vi "sort_scan_settings.vi"(7 "Scan settings array":T1[](array[typedef]) {"Enable display" items=["False", "True"]; "Current range" items=["Auto", "1 uA", "10 uA", "100 uA", "1 mA", "10 mA", "100 mA", "1 A"]; "Integration time (ms)" min=0.2; "Auto settling delay" items=["False", "True"]; "Sweep mode" items=["Staircase", "Pulsed"]; "Electrode configuration" items=["2-wire", "4-wire"]; "Logarithmic sweep" items=["False", "True"]; "Repeat scans" items=["False", "True"]; "No. of repeat scans" min=1.0 step=1.0; "Stabilisation mode" items=["V", "I"]; "Dual sweep" items=["False", "True"]; "Settling delay (ms)" min=0.0}, 10 "Setting name array":string[](array[string])) -> (0 "Sorted settings array":T1[](array[typedef]) {"Enable display" items=["False", "True"]; "Current range" items=["Auto", "1 uA", "10 uA", "100 uA", "1 mA", "10 mA", "100 mA", "1 A"]; "Integration time (ms)" min=0.2; "Auto settling delay" items=["False", "True"]; "Sweep mode" items=["Staircase", "Pulsed"]; "Electrode configuration" items=["2-wire", "4-wire"]; "Logarithmic sweep" items=["False", "True"]; "Repeat scans" items=["False", "True"]; "No. of repeat scans" min=1.0 step=1.0; "Stabilisation mode" items=["V", "I"]; "Dual sweep" items=["False", "True"]; "Settling delay (ms)" min=0.0}, 3 "Sorted name array":string[](array[string]))   [LabVIEW 2016]
uses:
  TypeDefs/settings.ctl
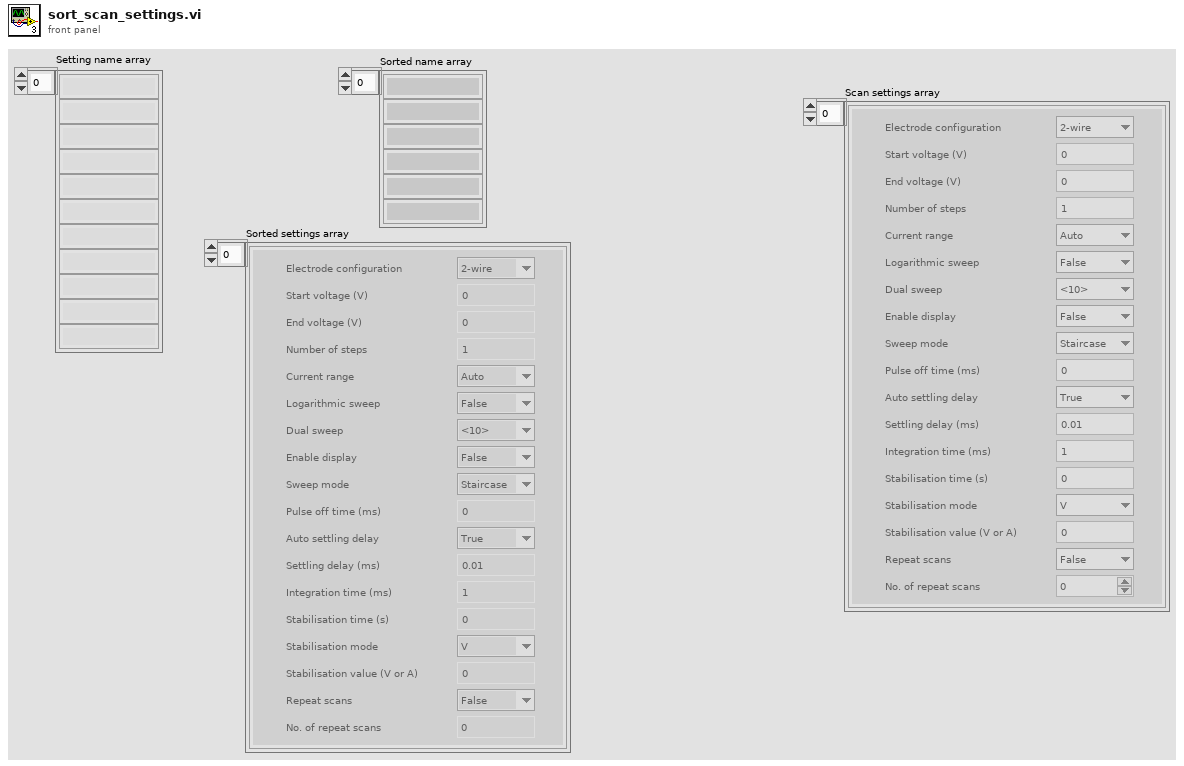
[diagram p1: front panel]
types:
  T1 = typedef "settings.ctl" = cluster{"Start voltage (V)":dbl, "End voltage (V)":dbl, "Number of steps":u32, "Settling delay (ms)":dbl, "Dual sweep":u16, "Stabilisation time (s)":dbl, "Stabilisation mode":u16, "Stabilisation value (V or A) ":dbl, "No. of repeat scans":dbl, "Repeat scans":u16, "Logarithmic sweep":u16, "Electrode configuration":u16, "Sweep mode":u16, "Auto settling delay":u16, "Pulse off time (ms)":dbl, "Integration time (ms)":dbl, "Current range":u16, "Enable display":u16}
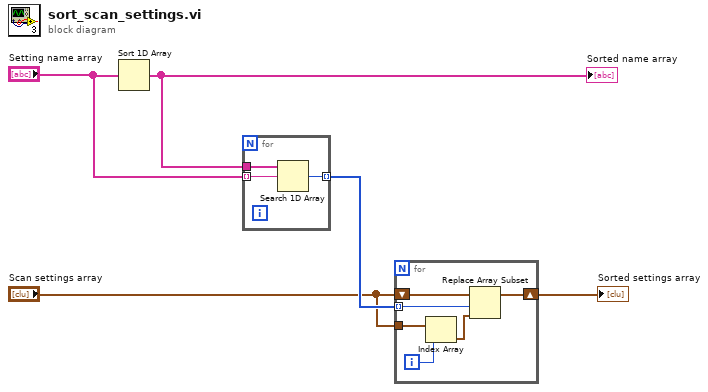
[diagram p0: block diagram]
diagram:
  n1 = Sort 1D Array(array="Setting name array") -> (sorted array=w5:string[])
  "Sorted name array" <- w5
  n2 = for {
    tunnel: w5 -> [w8]
    tunnel: "Setting name array" -> [w7] mode=indexing
    tunnel: [w6] -> w3 mode=indexing
    n3 = Search 1D Array(1D array=w8, element=w7) -> (index of element=w6:i32)  [unwired: 1 in]
  }
  n4 = for {
    shift-right: [w13] -> w2
    shift-left: "Scan settings array" -> [w14]
    tunnel: "Scan settings array" -> [w12]
    tunnel: w3 -> [w10] mode=indexing
    i -> [w9]
    n5 = Index Array(array=w12, index=w9) -> (element=w11:T1)
    n6 = Replace Array Subset(array=w14, new element=w11, index=w10) -> (w13:T1[])
  }
  "Sorted settings array" <- w2
